vi "CRYHardware Mic End.vi"   [LabVIEW 2013]
panel:
  # "Hardware Microphone Apply End Processing"
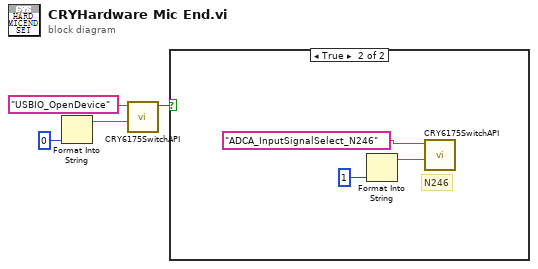
[diagram p0: block diagram]
diagram:
  n1 = Format Into String(0) -> (resulting string=w2:string)  [unwired: 3 in, 1 out]
  n2 = call "CRY6175SwitchAPI.vi"("Parameter"=w2, "Function Name"="USBIO_OpenDevice") -> ("bResult"=w1:bool)  [unwired: 9 in]
  n3 = case shown="True" w1 {
    frame False {
    }
    frame True {
      # "N246"
      n4 = Format Into String(u16 1 ("In Channel 1")) -> (resulting string=w5:string)  [unwired: 3 in, 1 out]
      n5 = call "CRY6175SwitchAPI.vi"("Parameter"=w5, "Function Name"="ADCA_InputSignalSelect_N246") -> ()  [unwired: 9 in, 1 out]
    }
  }
